vi "Prog1.vi"() -> ()   [LabVIEW 2021]
panel:
  out "length":i32
  out "String 3":string
  out "String 2":string
  out "String":string
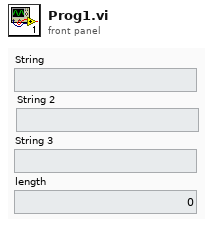
[diagram p1: front panel]
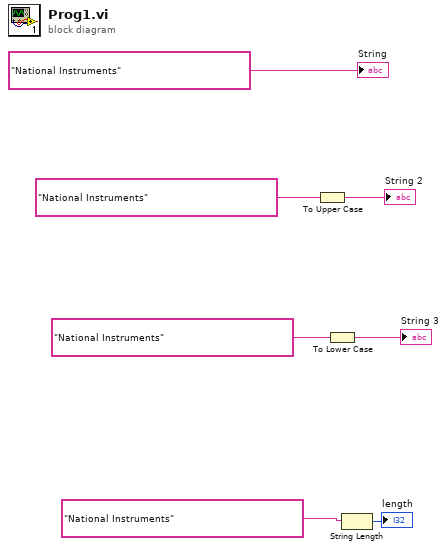
[diagram p0: block diagram]
diagram:
  n1 = To Upper Case(1:"National Instruments") -> (0:→"String 2":string)
  n2 = To Lower Case(string="National Instruments") -> (all lower case string=→"String 3":string)
  n3 = String Length(string="National Instruments") -> (length=→"length":i32)
  "String" <- "National Instruments"
